vi "CRYPeak index find.vi"(9 "Y array":dbl[](array[numeric]) format="%.2f", 10 "X array":dbl[](array[numeric]) format="%.2f", 11 "X value":dbl format="%.2f") -> (2 "Peak index of array":i32, 3 "X of peak point":dbl format="%.2f")   [LabVIEW 2013]
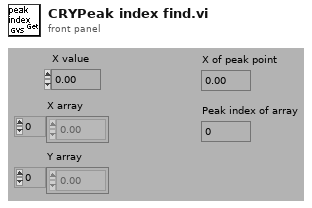
[diagram p1: front panel]
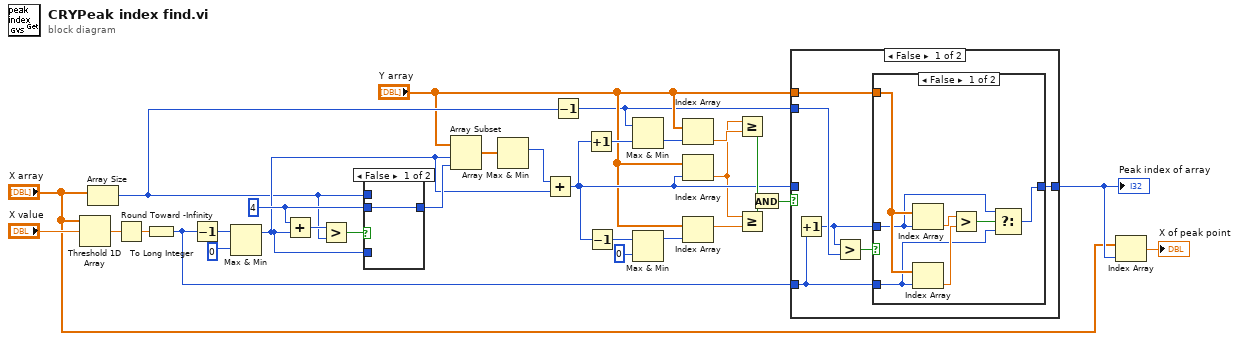
[diagram p0: block diagram]
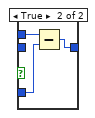
[diagram p4: hidden frame]
diagram:
  w27 = 4
  n1 = Threshold 1D Array(2:"X value", 3:"X array") -> (0:w7:dbl)  [unwired: 1 out]
  n2 = Array Size(array="X array") -> (size(s)=w17:i32)
  n3 = Round Toward -Infinity(1:w7) -> (0:w31:dbl)
  n4 = To Long Integer(number=w31) -> (32bit integer=w6:i32)
  n5 = Decrement(x=w6) -> (x-1=w9:i32)
  n6 = Max & Min(x=w9, y=0) -> (max(x,y)=w24:i32)  [unwired: 1 out]
  n7 = Add(x=w27, y=w24) -> (x+y=w28:i32)
  n8 = Greater?(x=w28, y=w17) -> (0:w29:bool)
  n9 = case shown="False" w29 {
    tunnel: w24 -> [_ w34]
    tunnel: w17 -> [_ w35]
    tunnel: [w32 w33] -> w26
    tunnel: w27 -> [w32 _]
    frame False {
    }
    frame True {
      n10 = Subtract(x=w35, y=w34) -> (x-y=w33:i32)
    }
  }
  n11 = Array Subset(array="Y array", index=w24, length=w26) -> (w25:dbl[])
  n12 = Array Max & Min(array=w25) -> (max index (indices)=w23:i32)  [unwired: 3 out]
  n13 = Add(x=w23, y=w24) -> (x+y=w11:i32)
  n14 = Decrement(x=w17) -> (x-1=w4:i32)
  n15 = Increment(x=w11) -> (x+1=w19:i32)
  n16 = Decrement(x=w11) -> (x-1=w21:i32)
  n17 = Max & Min(x=w4, y=w19) -> (min(x,y)=w18:i32)  [unwired: 1 out]
  n18 = Max & Min(x=w21, y=0) -> (max(x,y)=w20:i32)  [unwired: 1 out]
  n19 = Index Array(array="Y array", index=w18) -> (element=w15:dbl)
  n20 = Index Array(array="Y array", index=w11) -> (element=w10:dbl)
  n21 = Index Array(array="Y array", index=w20) -> (element=w16:dbl)
  n22 = Greater Or Equal?(x=w10, y=w15) -> (x >= y?=w14:bool)
  n23 = Greater Or Equal?(x=w10, y=w16) -> (x >= y?=w13:bool)
  n24 = And(x=w14, y=w13) -> (x .and. y?=w12:bool)
  n25 = case shown="False" w12 {
    tunnel: w11 -> [_ w50]
    tunnel: [w36 w50] -> w3
    tunnel: w6 -> [w38 _]
    tunnel: "Y array" -> [w37 _]
    tunnel: w4 -> [w41 _]
    frame False {
      n26 = Increment(x=w38) -> (x+1=w39:i32)
      n27 = Greater?(x=w39, y=w41) -> (0:w40:bool)
      n28 = case shown="False" w40 {
        tunnel: w39 -> [w44 _]
        tunnel: w38 -> [w43 w49]
        tunnel: w37 -> [w48 _]
        tunnel: [w42 w49] -> w36
        frame False {
          n29 = Index Array(array=w48, index=w44) -> (element=w47:dbl)
          n30 = Index Array(array=w48, index=w43) -> (element=w46:dbl)
          n31 = Greater?(x=w47, y=w46) -> (0:w45:bool)
          n32 = Select(t=w44, s=w45, f=w43) -> (s? t:f=w42:i32)
        }
        frame True {
        }
      }
    }
    frame True {
    }
  }
  "Peak index of array" <- w3
  n33 = Index Array(array="X array", index=w3) -> (element=→"X of peak point":dbl)
